vi "AlazarFFTSetWindowFunction.vi"(0 "DSP Handle":u64, 5 "Samples per record":u32, 7 "Real window array":sgl[](array[numeric]), 9 "Imag window array":sgl[](array[numeric]), 11 "error in (no error)":errorcluster) -> (4 "DSP Handle":u64, 15 "error out":errorcluster)   [LabVIEW 2018]
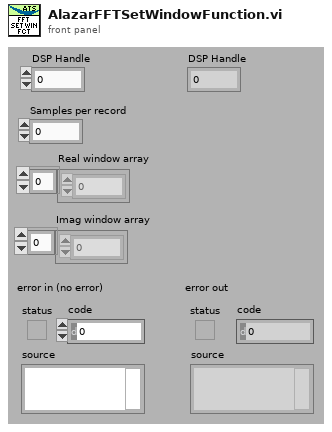
[diagram p1: front panel]
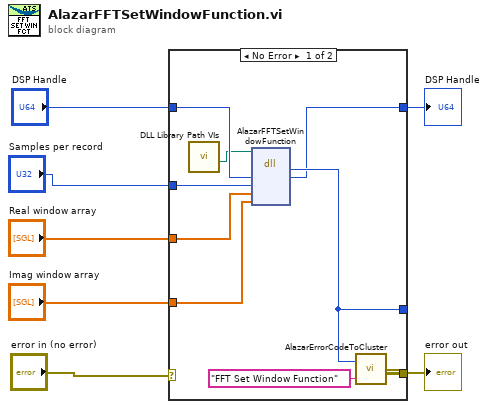
[diagram p0: block diagram]
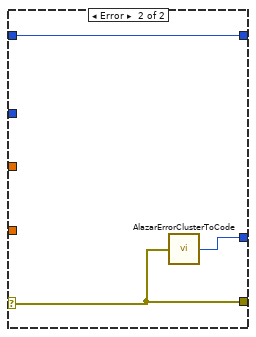
[diagram p2: hidden frame]
diagram:
  n1 = case shown="No Error" "error in (no error)" {
    selector: "error in (no error)" -> [_ w19]
    tunnel: [w13 w19] -> w6
    tunnel: [w15 w18] -> _
    tunnel: "DSP Handle" -> [w16 w17]
    tunnel: [w12 w17] -> w4
    tunnel: "Samples per record" -> [w11 _]
    tunnel: "Imag window array" -> [w10 _]
    tunnel: "Real window array" -> [w9 _]
    frame No Error {
      n2 = call "DLL Library Path VIs.vi"() -> ("Alazar"=w8:path)  [unwired: 5 in, 6 out]
      n3 = dll-call lib="C:/Project/SerialSectOCT - FFT GPU/SerialSectOCT/Labview Software/DLL/ATSApi.dll" fn="AlazarFFTSetWindowFunction"(path in=w8, "handle"=w16, "samplesPerRecord"=w11, "realWindowArray"=w9, "imagWindowArray"=w10) -> ("return type"=w15:u32, "handle"=w12:u64)  [unwired: 5 in, 2 out]
      n4 = call "AlazarErrorCodeToCluster.vi"("Message"="FFT Set Window Function", "Error Code"=w15) -> ("error out"=w13:errorcluster)
    }
    frame Error {
      n5 = call "AlazarErrorClusterToCode.vi"("error in (no error)"=w19) -> ("Error Code"=w18:u32)
    }
  }
  "DSP Handle" <- w4
  "error out" <- w6
